vi "Example_AOU_AWG_Secuence_from_file.vi"() -> ()   [LabVIEW 2013]
uses:
  <vilib>/Signadyne/Wave/base/waveformLoadWave.vi
panel:
  in  "Waveform file":string
  in  "AWG":u32
  in  "Run":bool
  out "errorOut":errorcluster
  in  "Close":bool
  in  "Prescaler":u32
  in  "Cycles":u32
  in  "Start Delay":u32
  in  "Trigger Mode":T1(ring)
  in  "nSlot":i32=7
  in  "nChassis":i32=1
  in  "partNumber":string="SD-PXE-AOU-H0002-128"
  # "Module Under Test"
  # "AWG Parameters"
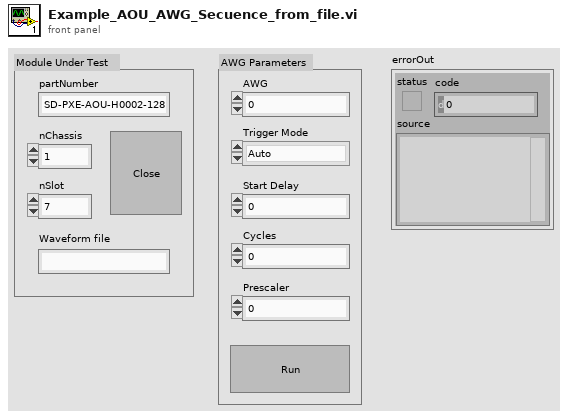
[diagram p1: front panel]
types:
  T1 = enum32{"Auto", "VI/HVI Trigger", "External Trigger"}
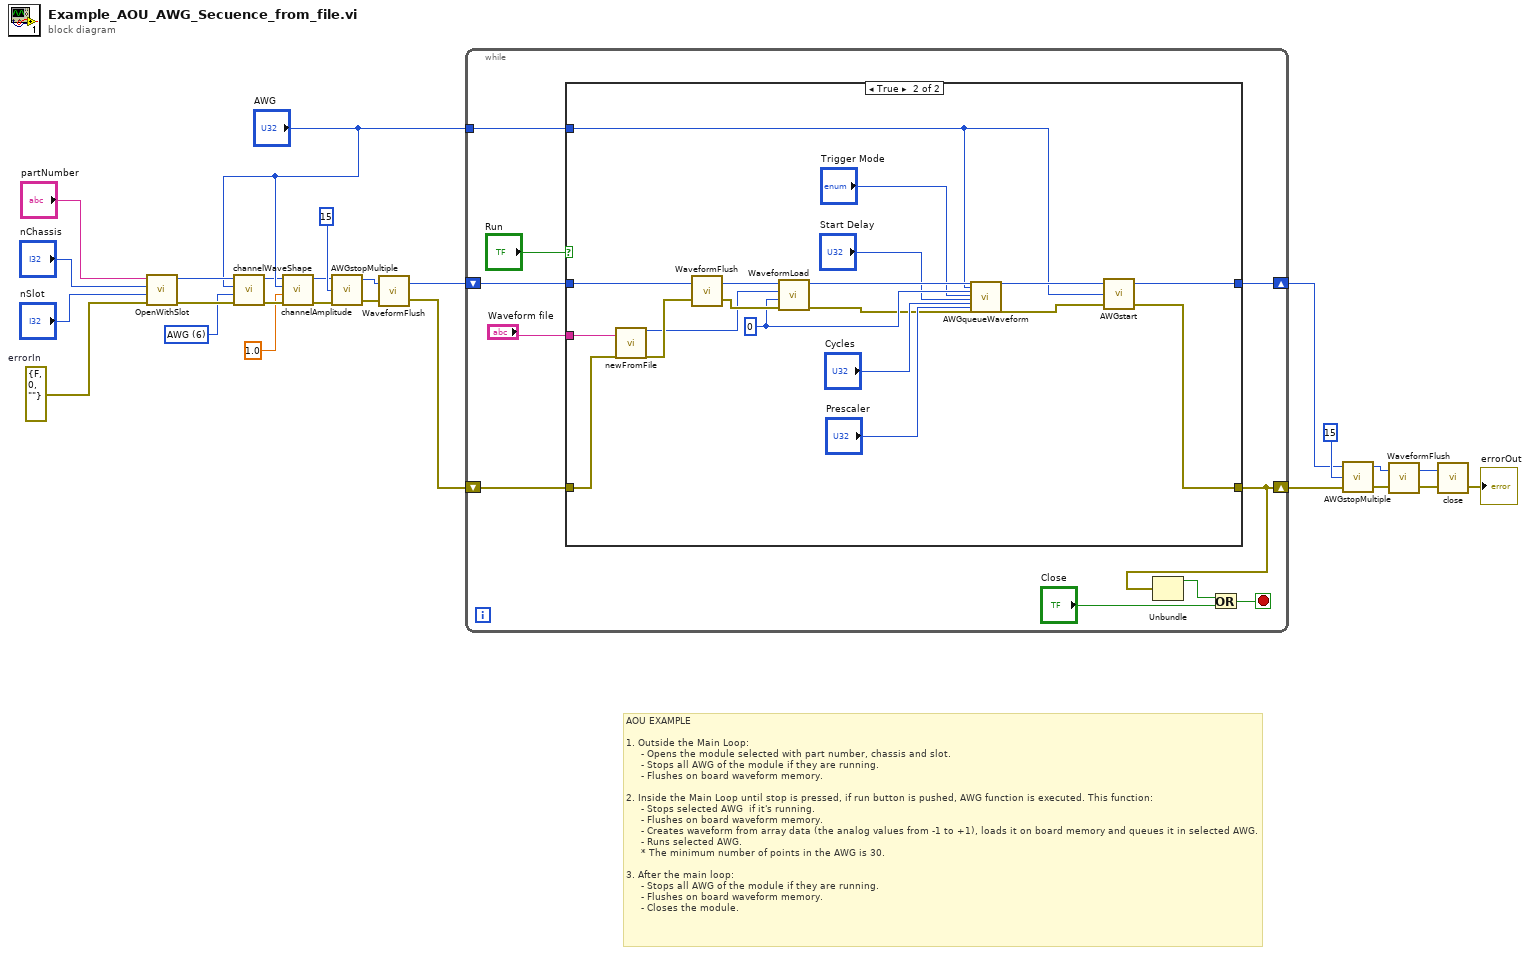
[diagram p0: block diagram]
diagram:
  w7 = 6 items=["None"=-1, "Sinusoidal"=1, "Triangular"=2, "Sawtooth"=3, "Square"=4, "DC"=5, "AWG"=6] ("waveShape")
  w11 = errorcluster {"status"=FALSE, "code"=0, "source"=""}  # errorIn
  # "AOU EXAMPLE\n\n1. Outside the Main Loop:\n     - Opens the module selected with part number, chassis and slot.\n     - Stops all AWG of the module if they are running.\n     - Flushes on board waveform memory.\n\n2. Inside the Main Loop until stop is pressed, if run button is pushed, AWG function is executed. This function:\n     - Stops selected AWG  if it's running.\n     - Flushes on board waveform memory.\n     - Creates waveform from array data (the analog values from -1 to +1), loads it on board memory and queues it in selected AWG.\n     - Runs selected AWG.\n     * The minimum number of points in the AWG is 30.  \n\n3. After the main loop:\n     - Stops all AWG of the module if they are running.\n     - Flushes on board waveform memory.\n     - Closes the module."
  n1 = call <vilib>:"OpenWithSlot.vi"("errorIn"=w11, "nSlot"="nSlot", "nChassis"="nChassis", "partNumber"="partNumber") -> ("errorOut"=w8:errorcluster, "moduleID"=w9:i32)  [unwired: 2 in]
  n2 = call <vilib>:"channelWaveShape.vi"("errorIn"=w8, "waveShape"=w7, "nChannel"="AWG", "moduleID"=w9) -> ("errorOut"=w6:errorcluster, "moduleIDOut"=w3:i32)  [unwired: 2 in]
  n3 = call <vilib>:"channelAmplitude.vi"("errorIn"=w6, "amplitude"=1.0, "nChannel"="AWG", "moduleID"=w3) -> ("errorOut"=w5:errorcluster, "moduleIDOut"=w2:i32)  [unwired: 2 in]
  n4 = call <vilib>:"AWGstopMultiple.vi"("errorIn"=w5, "AWGmask"=15, "moduleID"=w2) -> ("errorOut"=w14:errorcluster, "moduleIDOut"=w13:i32)  [unwired: 1 in]
  n5 = call <vilib>:"WaveformFlush.vi"("errorIn"=w14, "moduleID"=w13) -> ("errorOut"=w23:errorcluster, "moduleIDOut"=w24:i32)
  n6 = while {
    shift-right: [w30] -> w18
    shift-left: w23 -> [w27]
    shift-right: [w34] -> w10
    shift-left: w24 -> [w36]
    tunnel: "AWG" -> [w29]
    stop <- w33 stop-if-true
    n7 = case shown="True" "Run" {
      tunnel: w36 -> [w38 w54]
      tunnel: w27 -> [w37 w57]
      tunnel: [w37 w39] -> w30
      tunnel: [w38 w40] -> w34
      tunnel: w29 -> [_ w41]
      tunnel: "Waveform file" -> [_ w56]
      frame False {
      }
      frame True {
        w49 = 0 ("waveformNumber")
        n8 = call <vilib>:"newFromFile.vi"("waveformFile"=w56, "errorIn"=w57) -> ("waveformID"=w51:i32, "errorOut"=w55:errorcluster)  [unwired: 16 in]
        n9 = call <vilib>:"WaveformFlush.vi"("errorIn"=w55, "moduleID"=w54) -> ("errorOut"=w52:errorcluster, "moduleIDOut"=w53:i32)
        n10 = call-poly <vilib>:"WaveformLoad.vi"("errorIn"=w52, "waveformNumber"=w49, "waveformID"=w51, "moduleID"=w53) -> ("errorOut"=w44:errorcluster, "moduleIDOut"=w50:i32)  [unwired: 3 in, 1 out]
        n11 = call <vilib>:"AWGqueueWaveform.vi"("moduleID"=w50, "nAWG"=w41, "waveformNumber"=w49, "triggerMode"="Trigger Mode", "startDelay"="Start Delay", "cycles"="Cycles", "prescaler"="Prescaler", "errorIn"=w44) -> ("moduleIDOut"=w42:i32, "errorOut"=w43:errorcluster)  [unwired: 18 in]
        n12 = call <vilib>:"AWGstart.vi"("errorIn"=w43, "nAWG"=w41, "moduleID"=w42) -> ("errorOut"=w39:errorcluster, "moduleIDOut"=w40:i32)  [unwired: 1 in]
      }
    }
    n13 = Unbundle(w30) -> ("status"=w32:bool)  [unwired: 2 out]
    n14 = Or(x=w32, y="Close") -> (x .or. y?=w33:bool)
  }
  n15 = call <vilib>:"AWGstopMultiple.vi"("errorIn"=w18, "AWGmask"=15, "moduleID"=w10) -> ("errorOut"=w17:errorcluster, "moduleIDOut"=w16:i32)  [unwired: 1 in]
  n16 = call <vilib>:"WaveformFlush.vi"("errorIn"=w17, "moduleID"=w16) -> ("errorOut"=w21:errorcluster, "moduleIDOut"=w20:i32)
  n17 = call <vilib>:"close.vi"("errorIn"=w21, "moduleID"=w20) -> ("errorOut"=→"errorOut":errorcluster)  [unwired: 1 in]
